vi "Roller Loop.vi"   [LabVIEW 2014]
uses:
  Common Code/Roller Indicators.ctl
  Common Code/Roller Mode Enum.ctl
  Common Code/Auto Roller Commands.ctl
  Common Code/Inner Roller States.ctl
  Sensors/Pot Data.ctl
  Untip Can States.ctl
  Roller Modes.ctl
  Really Real Manual Align.ctl
  Common Code/Change Detect Int.vi
  Robot Global Data.vi
  <vilib>/Rock Robotics/WPI/Solenoid/Deprecated/WPI_SolenoidSetBool.vi
types:
  T1 = typedef "Roller Modes.ctl" = cluster{"Auto Roller Command":T2, "Roller Mode":T3, "Override Intake Speed":dbl}
  T2 = typedef "Auto Roller Commands.ctl" = enum16{"Drag Tote", "Grab Tote", "Idle", "Eject Tote", "Untip Can", "Grab Can"}
  T3 = typedef "Roller Mode Enum.ctl" = enum16{"Manual", "Safe", "Auto"}
  T4 = typedef "Inner Roller States.ctl" = enum16{"Turn Tote Portrait", "Acquire Tote", "Absorb Tote", "Turn Tote Right", "Turn Tote Left", "Acquire Can", "Absorb Can", "Turn Can", "Hold Tote"}
  T5 = typedef "Roller Indicators.ctl" = cluster{"Rollers Closed?":bool, "Roller Mode":T3, "Auto Roller State":T2, "Tote Inside?":bool, "Intake State":T4, "Left Ping Dist":sgl, "Right Ping Dist":sgl, "Potentiometer Cluster":T6, "PING Decision":T4, "Left Arm Closed?":bool, "Portrait?":bool, "Right Arm Closed?":bool, "Left Out":sgl, "Right Out":sgl, "Left Current":sgl, "Right Current":sgl, "Tote Load Complete?":bool, "Untip Complete?":bool, "Untip State":T7, "Roller Safety Open":bool}
  T6 = typedef "Pot Data.ctl" = cluster{"Left Pot Zero":sgl, "Right Pot Zero":sgl, "Left Potentiometer":sgl, "Right Potentiometer":sgl, "Left Pot Non Zero":sgl, "Right Pot Non Zero":sgl}
  T7 = typedef "Untip Can States.ctl" = enum16{"Release Can", "Catch Can", "Idle"}
  T8 = typedef "Dashboard Control Data.ctl" = cluster{"Cam Exposure":dbl, "Go to angle":dbl, "Steer PID Gains":cluster{"proportional gain (Kc)":dbl, "integral time (Ti, min)":dbl, "derivative time (Td, min)":dbl}, "Steer PID output Range":cluster{"output high":dbl, "output low":dbl}, "Pressure m \nValue":dbl, "Pressure b \nValue":dbl, "Roller Command Cluster ":T9, "Elevator":T10, "Encoder Control":T12, "Auton Settings":cluster{"Drive Dist Window Size":dbl}, "Drivetrain Settings":T13, "Lance":T14}
  T9 = typedef "Roller Control.ctl" = cluster{"Intake Speed":dbl, "Turn In Speed":dbl, "Unload Speed":dbl, "Turn Out Speed":dbl, "Ping Align Tolerance":dbl, "Tote Range Threshold":dbl, "Right Pot 0":dbl, "Pot Threshold":dbl, "Left Pot 0":dbl, "Right Pot Scale":dbl, "Left Pot Scale":dbl, "Min Elevator Height":dbl, "Eject Time":dbl, "Eject US Threshold":dbl, "Anti-Twitch Time":u32, "Ping Caring Threshold":dbl, "Pot Diff Threshold":dbl, "Pinch Sustain":u32, "Absorb Give Up Threshold":dbl, "Untip In Threshold":dbl, "Untip Grab Range":dbl, "Ultrasonic Hold Time":u32, "Landscape Absorb Time":u32, "Pot Use Wait Time":u32, "Can Turn Stop Range":dbl, "HP Load Speed":dbl, "Stick Multiplier":dbl, "Coop Eject Speed":dbl}
  T10 = typedef "Elevator DB Control.ctl" = cluster{"PID Output Range":cluster{"output high":dbl, "output low":dbl}, "PID gains":cluster{"proportional gain (Kc)":dbl, "integral time (Ti, min)":dbl, "derivative time (Td, min)":dbl}, "Height Tolerance":sgl, " Encoder Constant":dbl, "Eject Time":sgl, "Zeroing Speed":sgl, "Presets":T11, "Ping Detect Threshold":sgl, "Trashcan Detect Threshold":sgl, "Zero Filter Time":dbl, "Stabilizer Open Time":dbl, "Zero Creep Speed":dbl, "Max Current":dbl, "Current Trip Time":dbl, "Abort Pitch":dbl, "Finger m":dbl, "Finger b":dbl, "Finger max ":dbl, "Finger Stabilizer":dbl, "Finger Store":dbl, "Finger Stop Store":dbl, "Stabilizer Close Time":dbl, "Finger min":dbl, "Unstick gain":dbl, "Full Detect Max":dbl}
  T11 = typedef "Elevator Presets.ctl" = cluster{"Pickup 2 w/ Tote":sgl, "Pickup 2 w/ Trashcan":sgl, "Pickup 3 w/ Tote":sgl, "Pickup 3 w/ Trashcan":sgl, "Bottom":sgl, "Pickup 1 w/ Tote":sgl, "Pickup Trashcan":sgl, "Pickup 1 w/ Trashcan":sgl, "Eject":sgl, "Hold Low":sgl, "Step add height":sgl, "Untip Lift":dbl, "Drop Stack":dbl, "HP Load Hold":dbl, "HP Load Drop":dbl, "HP Load Hold Can":dbl, "Store can max":dbl, "HP Drag Score":dbl, "HP Drag Finish":dbl, "Finger trashcan avoid":dbl, "Full":dbl}
  T12 = typedef "Encoder Control.ctl" = cluster{"Left Tick Constant":dbl, "Right Tick Constant":dbl, "Center Tick Constant":dbl, "Reset?":bool, "Y Dist":cluster{"PID gains":cluster{"proportional gain (Kc)":dbl, "integral time (Ti, min)":dbl, "derivative time (Td, min)":dbl}}, "X Dist":cluster{"PID gains":cluster{"proportional gain (Kc)":dbl, "integral time (Ti, min)":dbl, "derivative time (Td, min)":dbl}}, "Y Stop Thresh":dbl, "Y Stop Speed":dbl, "X Stop Thresh":dbl, "X Stop Speed":dbl}
  T13 = typedef "Drivetrain Settings.ctl" = cluster{"Gyro Tolerance":sgl, "Strafe Correct max steer":sgl, "Strafe Timer Wait":sgl, "Throttle Ramp (ms)":sgl, "Strafe Ramp (ms)":sgl, "Angular rate compensation":bool, "Throttle to Rate Scale":sgl, "Rate compensation gain":sgl, "Creep Steer":sgl, "Creep Throttle":sgl}
  T14 = typedef "Pike DB Controls.ctl" = cluster{"Down Speed":dbl, "Up Speed":dbl, "Max Down Time":dbl, "Max Up Time":dbl, "Current Limit":dbl}
  T15 = typedef "Ultrasonic Indicators.ctl" = cluster{"Left Distance":dbl, "Right Distance":dbl, "Center Distance":dbl, "Left Distance Unfilter":dbl, "Right Distance Unfilter":dbl, "Center Distance Unfilter":dbl}
  T16 = typedef "Roller Manual Bools.ctl" = cluster{"Manual Claw":bool, "Manual Align":T17, "Left Speed":dbl, "Right Speed":dbl}
  T17 = typedef "Really Real Manual Align.ctl" = enum16{"In", "Left", "Right", "Out", "Idle", "HP Load", "Speeds"}
  T18 = typedef "Elevator Status.ctl" = cluster{"Height":dbl, "Enc Value":dbl, "Limit Override":bool, "Mode":T19, "High IR":bool, "Motor Out":dbl, "Ping Detect":bool, "Auto Elevator Indicators":T20, "Master Current":dbl, "Slave Current":dbl, "High Current":bool, "Current Tripped":bool, "Top Limit":bool, "Bottom Limit":bool, "Eject Piston":bool, "Stabilizer":bool, "Finger":bool, "Finger Height":dbl, "Finger Raw":dbl, "Finger at Bottom":bool}
  T19 = typedef "Elevator Mode.ctl" = enum16{"Manual", "Safe", "Auto"}
  T20 = typedef "Auto Elevator Indicators.ctl" = cluster{"Target Out":dbl, "Storing Trashcan?":bool, "State":T21, "In Range":bool, "Store Can Command":bool, "HP Load":bool}
  T21 = typedef "Elevator State.ctl" = enum16{"Idle", "Goto Load Position", "Wait for Load", "Load Drop", "Load Lift", "Drop Stack", "Goto Eject Position", "Eject ", "Raise Trashcan", "Open Stabilizer", "Untip Drop", "Untip Wait", "Untip Lift", "Abort Load", "HP Load Wait", "HP Load Drop", "HP Load Lift", "HP Load Abort", "Close Stabilizer", "HP Load Unfinish", "HP Load Score", "HP Load Finish", "HP Goto Finish Down", "HP Goto Finish Up", "Full"}
  T22 = typedef "WPI_MotorControlDeviceRef.ctl" = cluster{"DeviceStatus":errorcluster, "Type":T23, "PWM":cluster{"Controller":T24, "PWM Channel":T25, "DeadBand":T26}, "CAN":cluster{"Device Number":u8, "Control Mode":T27, "Semaphore":T28, "Max Vout":dbl, "TalonSRX Control Mode":T29}, "Invert":bool, "TransformRef":T30, "InvTransformRef":T30}
  T23 = typedef "WPI_MotorControlType.ctl" = enum16{"PWM", "CAN", "CANTalonSRX"}
  T24 = typedef "FPGA_TypedefDigitalModule.ctl" = enum16{"Controller 1"}
  T25 = typedef "FPGA_DIOPWMChannel.ctl" = enum8{"PWM 0", "PWM 1", "PWM 2", "PWM 3", "PWM 4", "PWM 5", "PWM 6", "PWM 7", "PWM 8", "PWM 9", "PWM MXP 0", "PWM MXP 1", "PWM MXP 2", "PWM MXP 3", "PWM MXP 4", "PWM MXP 5", "PWM MXP 6", "PWM MXP 7", "PWM MXP 8", "PWM MXP 9", "Invalid"}
  T26 = typedef "WPI_PWMDeadband.ctl" = cluster{"Name":string, "maxPositivePwm":i32, "minPositivePwm":i32, "centerPwm":i32, "maxNegativePwm":i32, "minNegativePwm":i32, "angularRange":u16}
  T27 = typedef "WPI_CANJaguar_ControlMode.ctl" = enum8{"Percent VBus", "Current", "Speed", "Position", "Voltage"}
  T28 = typedef "Semaphore RefNum" = refnum<k1>
  T29 = typedef "WPI_CANTalonSRX_APIControlMode.ctl" = enum8{"Percent VBus", "Speed", "Position", "Slave", "Unchanged / Invalid"}
  T30 = typedef "WPI_PWMTransform_ConPane.ctl" = refnum<vi>
  T31 = typedef "WPI_SolenoidDevRef.ctl" = cluster{"DevStatus":errorcluster, "Pneumatics Control Module":u8, "Forward Solenoid Channel":T32, "Reverse Solenoid Channel":T32}
  T32 = typedef "WPI_SolenoidChannel.ctl" = enum8{"Solenoid 0", "Solenoid 1", "Solenoid 2", "Solenoid 3", "Solenoid 4", "Solenoid 5", "Solenoid 6", "Solenoid 7", "Invalid"}
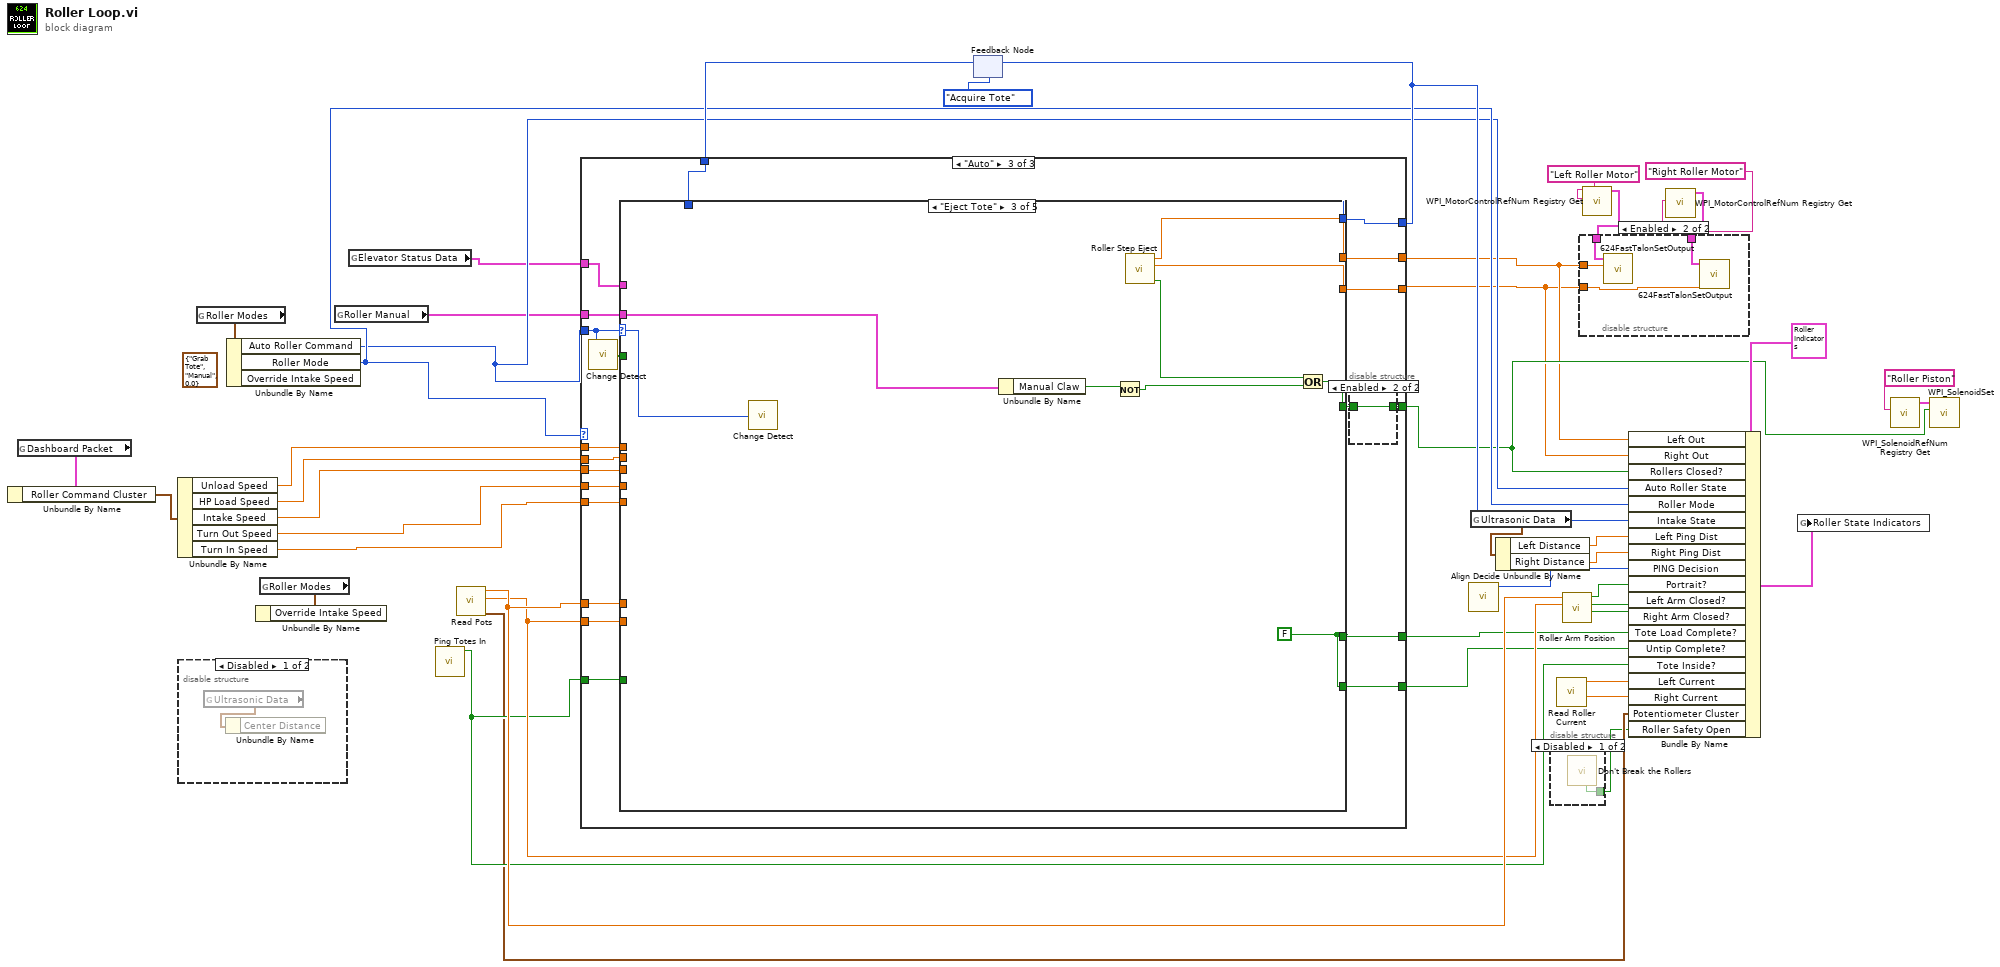
[diagram p0: block diagram]
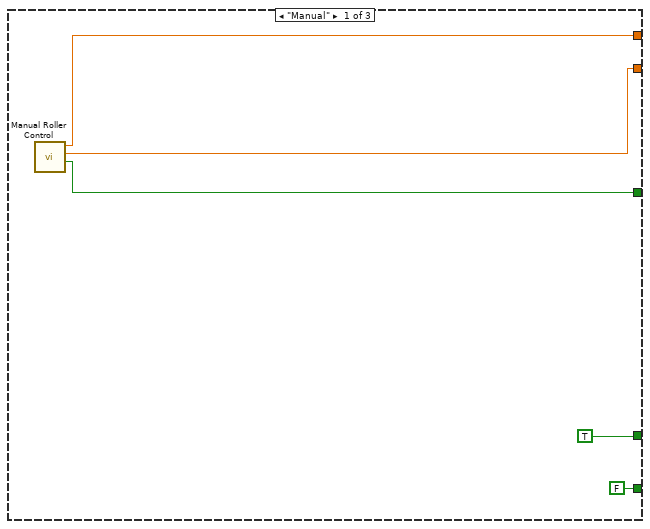
[diagram p3: hidden frame]
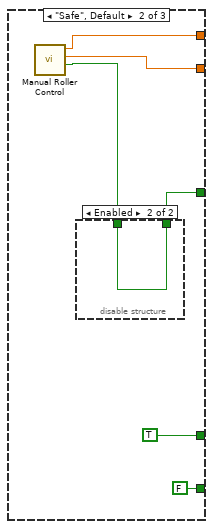
[diagram p4: hidden frame]
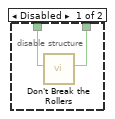
[diagram p5: hidden frame]
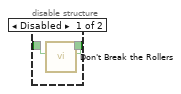
[diagram p6: hidden frame]
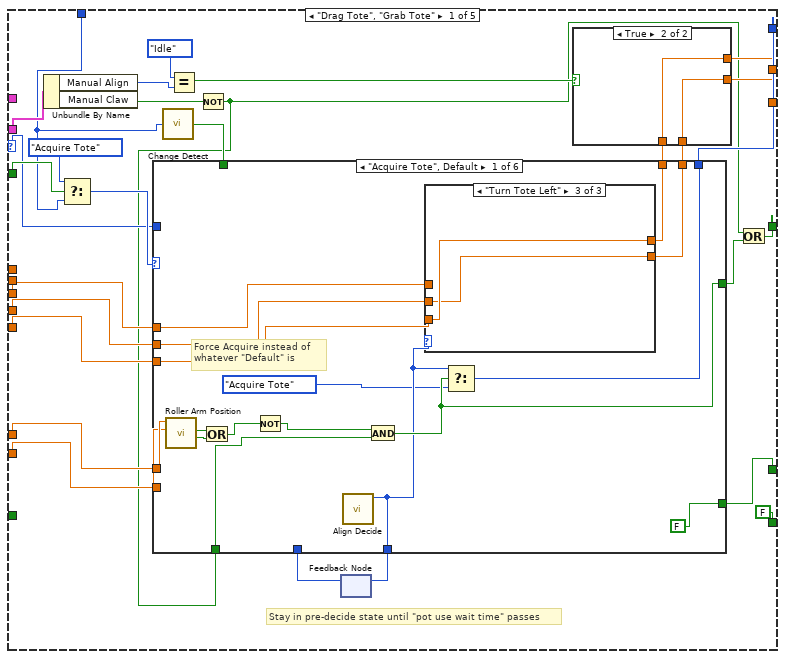
[diagram p7: hidden frame]
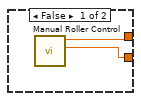
[diagram p8: hidden frame]
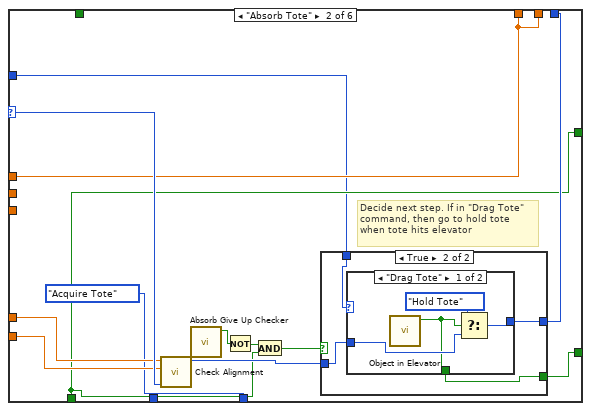
[diagram p11: hidden frame]
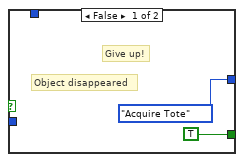
[diagram p12: hidden frame]
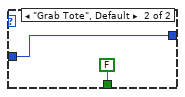
[diagram p13: hidden frame]
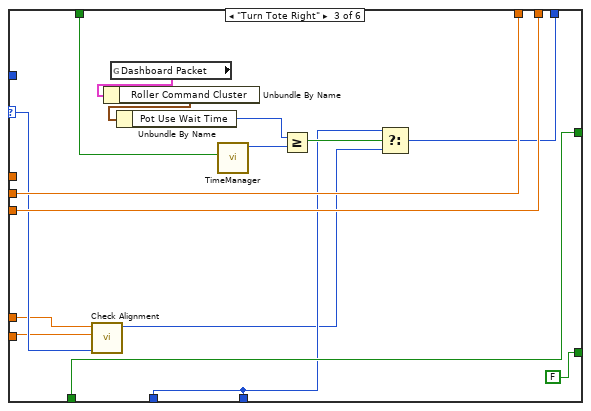
[diagram p14: hidden frame]
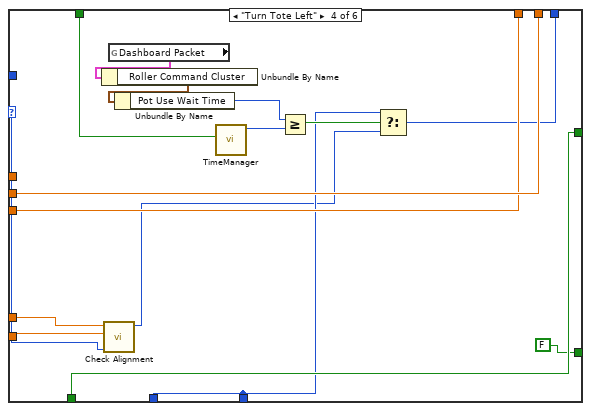
[diagram p15: hidden frame]
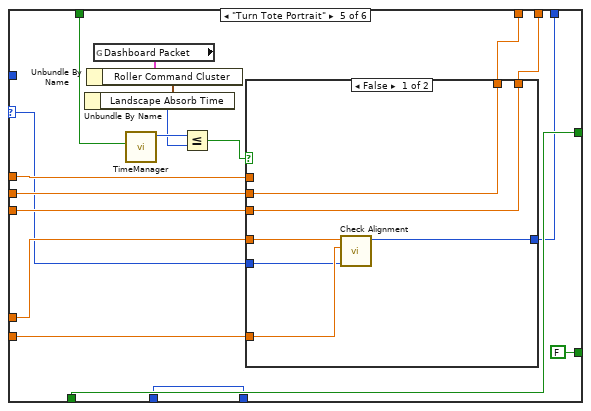
[diagram p16: hidden frame]
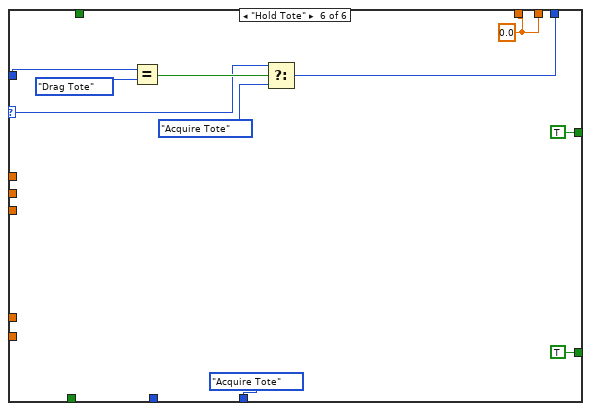
[diagram p18: hidden frame]
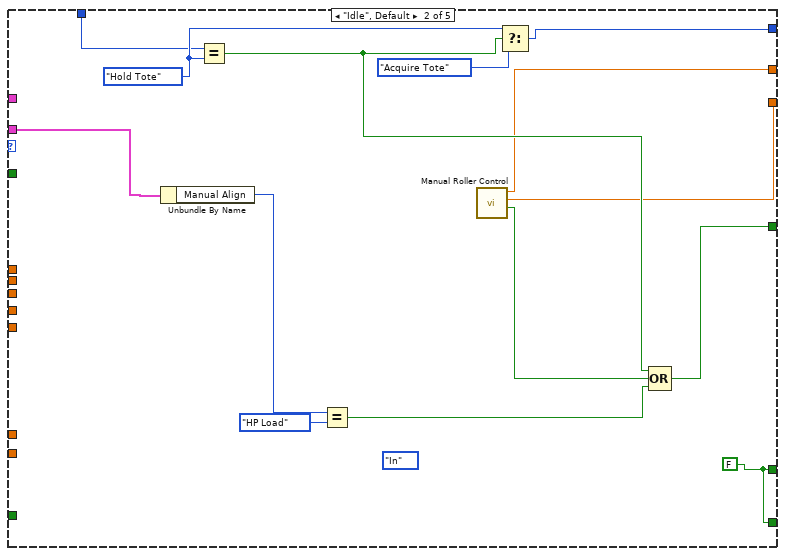
[diagram p19: hidden frame]
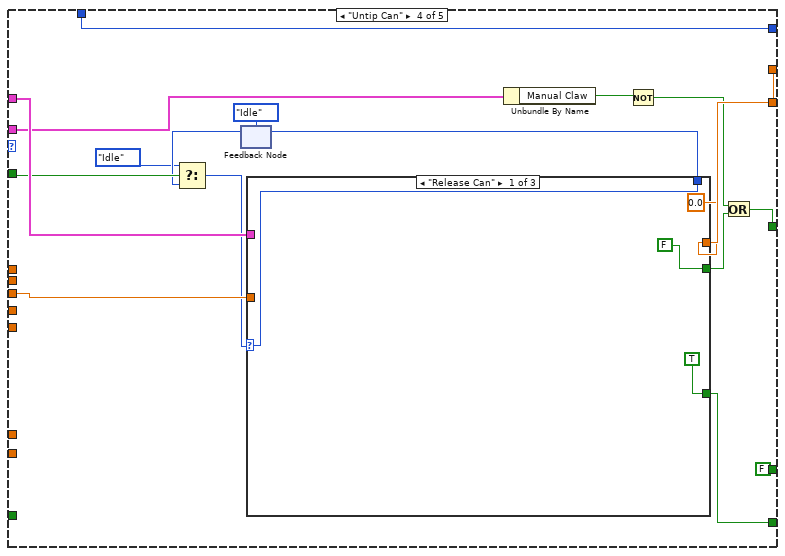
[diagram p20: hidden frame]
diagram:
  (unwired) T1 {"Auto Roller Command"=enum."Grab Tote", "Roller Mode"=enum."Manual", "Override Intake Speed"=0.0} ("input cluster")
  n1 = global read "Robot Global Data.vi" "Dashboard Packet"() -> (w24:T8)
  n2 = Unbundle By Name(w24) -> ("Roller Command Cluster"=w25:T9)
  n3 = Unbundle By Name(w25) -> ("Unload Speed"=w12:dbl, "HP Load Speed"=w4:dbl, "Intake Speed"=w11:dbl, "Turn Out Speed"=w2:dbl, "Turn In Speed"=w1:dbl)
  n4 = disable-structure shown="Disabled" {
    frame Disabled {
      n5 = global read "Robot Global Data.vi" "Ultrasonic Data"() -> (w44:T15)
      n6 = Unbundle By Name(w44) -> ()  [unwired: 1 out]
    }
    frame Enabled {
    }
  }
  n7 = global read "Robot Global Data.vi" "Roller Modes"() -> (w38:T1)
  n8 = Unbundle By Name(w38) -> ("Auto Roller Command"=w35:T2, "Roller Mode"=w36:T3)  [unwired: 1 out]
  n9 = global read "Robot Global Data.vi" "Roller Modes"() -> (w3:T1)
  n10 = Unbundle By Name(w3) -> ()  [unwired: 1 out]
  n11 = global read "Robot Global Data.vi" "Roller Manual"() -> (w20:T16)
  n12 = global read "Robot Global Data.vi" "Elevator Status Data"() -> (w21:T18)
  n13 = call "Ping Totes In.vi"() -> ("In?"=w10:bool)  [unwired: 11 in]
  n14 = call "Read Pots.vi"() -> ("Pot Write Cluster"=w7:T6, "Right Pot"=w28:dbl, "Left Pot"=w29:dbl)  [unwired: 7 in, 2 out]
  n15 = feedback #1(Inner_Roller_States."Acquire Tote" ("Enum")) -> (w42:T4)
  n16 = case shown="\"Auto\"" w36 {
    tunnel: w20 -> [_ _ w69]
    tunnel: w11 -> [_ _ w77]
    tunnel: w2 -> [_ _ w75]
    tunnel: w1 -> [_ _ w76]
    tunnel: w35 -> [_ _ w60]
    tunnel: [_ _ w73] -> w37
    tunnel: w42 -> [_ _ w78]
    tunnel: [w45 w55 w66] -> w33
    tunnel: w10 -> [_ _ w74]
    tunnel: [w47 w52 w72] -> w27
    tunnel: [w46 w51 w71] -> w26
    tunnel: w12 -> [_ _ w70]
    tunnel: w29 -> [_ _ w68]
    tunnel: w28 -> [_ _ w67]
    tunnel: [TRUE TRUE w64] -> w23
    tunnel: w21 -> [_ _ w63]
    tunnel: [FALSE FALSE w61] -> w22
    tunnel: w4 -> [_ _ w59]
    frame "Manual" {
      n17 = call "Manual Roller Control.vi"() -> ("Boolean"=w45:bool, "Right Speed Out"=w46:dbl, "Left Speed Out"=w47:dbl)  [unwired: 9 in]
    }
    frame "Safe", Default {
      n18 = call "Manual Roller Control.vi"() -> ("Boolean"=w50:bool, "Right Speed Out"=w51:dbl, "Left Speed Out"=w52:dbl)  [unwired: 9 in]
      n19 = disable-structure shown="Enabled" {
        disable-tunnel: [w57 w58] -> w55
        disable-tunnel: w50 -> [w56 w58]
        frame Disabled {
          n20 = call "Don't Break the Rollers.vi"("Rollers close in"=w56) -> ("Roller close out"=w57:bool)  [unwired: 9 in, 1 out]
        }
        frame Enabled {
        }
      }
    }
    frame "Auto" {
      n21 = call-poly "Change Detect.vi"("In"=w60) -> ("Changed?"=w62:bool)
      n22 = case shown="\"Eject Tote\"" w60 {
        selector: w60 -> [w85 _ w250 _ _]
        tunnel: w78 -> [w88 w237 w252 w267 w320]
        tunnel: [w84 w238 w247 w257 w302] -> w65
        tunnel: w77 -> [w109 _ _ w265 w316]
        tunnel: w76 -> [w108 _ _ _ w314]
        tunnel: w75 -> [w107 _ _ _ w315]
        tunnel: w74 -> [_ _ _ _ _]
        tunnel: [w97 w236 w252 w267 w311] -> w73
        tunnel: [w96 w231 w249 w260 w312] -> w72
        tunnel: [w93 w230 w248 w260 w313] -> w71
        tunnel: w70 -> [_ _ _ _ _]
        tunnel: w69 -> [w103 w242 w244 w254 w322]
        tunnel: w68 -> [w106 _ _ _ _]
        tunnel: w67 -> [w105 _ _ _ _]
        tunnel: [w104 w241 w251 FALSE FALSE] -> w64
        tunnel: w63 -> [_ _ _ w268 _]
        tunnel: w62 -> [w89 _ _ w264 w321]
        tunnel: [FALSE w241 w251 w259 FALSE] -> w61
        tunnel: w59 -> [_ _ _ _ _]
        frame "Drag Tote", "Grab Tote" {
          # "Stay in pre-decide state until \"pot use wait time\" passes"
          n23 = Unbundle By Name(w103) -> ("Manual Align"=w100:T17, "Manual Claw"=w102:bool)
          n24 = Select(t=Inner_Roller_States."Acquire Tote", s=w89, f=w88) -> (s? t:f=w86:T4)
          n25 = call-poly "Change Detect.vi"("In"=w88) -> ("Changed?"=w92:bool)
          n26 = Equal?(x=Really_Real_Manual_Align."Idle" ("y"), y=w100) -> (x = y?=w98:bool)
          n27 = Not(x=w102) -> (.not. x?=w82:bool)
          n28 = feedback #2() -> (w90:T4)  [unwired: 1 in]
          n29 = case shown="\"Acquire Tote\", Default" w86 {
            selector: w86 -> [_ w146 w174 w192 w198 w221]
            tunnel: w82 -> [w120 w140 w171 w187 w204 _]
            tunnel: [w119 w140 w171 w187 w204 TRUE] -> w83
            tunnel: [w130 w148 w161 w179 w197 w219] -> w97
            tunnel: w109 -> [w129 w143 _ _ w207 _]
            tunnel: w108 -> [w128 _ w176 w188 w201 _]
            tunnel: w107 -> [w127 _ w175 w189 w202 _]
            tunnel: [w126 w143 w175 w188 w206 w228] -> w95
            tunnel: [w125 w143 w176 w189 w205 w228] -> w94
            tunnel: w106 -> [w124 w145 w173 w191 w199 _]
            tunnel: w105 -> [w123 w144 w172 w190 w200 _]
            tunnel: [FALSE w142 FALSE FALSE FALSE TRUE ("Boolean")] -> w104
            tunnel: w92 -> [_ _ w167 w182 w210 _]
            tunnel: [w115 Inner_Roller_States."Acquire Tote" ("Next Step") w163 w181 w193 Inner_Roller_States."Acquire Tote" ("Next Step")] -> w91
            tunnel: w90 -> [_ _ w163 w181 w193 _]
            tunnel: w85 -> [_ w136 _ _ _ w224]
            frame "Acquire Tote", Default {
              # "Force Acquire instead of \nwhatever \"Default\" is"
              n30 = call "Roller Arm Position.vi"("Right Pot"=w123, "Left Pot"=w124) -> ("Right Closed?"=w122:bool, "Left Closed?"=w121:bool)  [unwired: 6 in, 2 out]
              n31 = Or(x=w121, y=w122) -> (x .or. y?=w118:bool)
              n32 = Not(x=w118) -> (.not. x?=w117:bool)
              n33 = call "Align Decide.vi"() -> ("Next Step"=w115:T4)  [unwired: 11 in]
              n34 = And(x=w117, y=w120) -> (x .and. y?=w119:bool)
              n35 = case shown="\"Turn Tote Left\"" w115 {
                tunnel: w129 -> [w131 _ _]
                tunnel: w128 -> [_ w133 w135]
                tunnel: w127 -> [_ w132 w134]
                tunnel: [w131 w132 w135] -> w126
                tunnel: [w131 w133 w134] -> w125
                frame "Absorb Tote", Default {
                }
                frame "Turn Tote Right" {
                }
                frame "Turn Tote Left" {
                }
              }
              n36 = Select(t=w115, s=w119, f=Inner_Roller_States."Acquire Tote") -> (s? t:f=w130:T4)
            }
            frame "Absorb Tote" {
              # "Decide next step. If in \"Drag Tote\"\ncommand, then go to hold tote\nwhen tote hits elevator"
              n37 = call "Check Alignment.vi"("Current State"=w146, "Right Pot"=w144, "Left Pot"=w145) -> ("State Output"=w147:T4)  [unwired: 8 in]
              n38 = call "Absorb Give Up Checker.vi"() -> ("Give Up?"=w141:bool)  [unwired: 11 in]
              n39 = Not(x=w141) -> (.not. x?=w139:bool)
              n40 = And(x=w139, y=w140) -> (x .and. y?=w138:bool)
              n41 = case shown="True" w138 {
                tunnel: [Inner_Roller_States."Acquire Tote" ("State Output") w152] -> w148
                tunnel: w147 -> [_ w153]
                tunnel: [TRUE w151] -> w142
                tunnel: w136 -> [_ w154]
                frame False {
                  # "Object disappeared"
                  # "Give up!"
                }
                frame True {
                  n42 = case shown="\"Drag Tote\"" w154 {
                    tunnel: w153 -> [w158 w160]
                    tunnel: [w157 w160] -> w152
                    tunnel: [w155 FALSE ("Boolean")] -> w151
                    frame "Drag Tote" {
                      n43 = call "Object in Elevator.vi"() -> ("Ping Detect"=w155:bool)  [unwired: 11 in]
                      n44 = Select(t=Inner_Roller_States."Hold Tote", s=w155, f=w158) -> (s? t:f=w157:T4)
                    }
                    frame "Grab Tote", Default {
                    }
                  }
                }
              }
            }
            frame "Turn Tote Right" {
              n45 = call "Check Alignment.vi"("Current State"=w174, "Right Pot"=w172, "Left Pot"=w173) -> ("State Output"=w162:T4)  [unwired: 8 in]
              n46 = global read "Robot Global Data.vi" "Dashboard Packet"() -> (w169:T8)
              n47 = Unbundle By Name(w169) -> ("Roller Command Cluster"=w168:T9)
              n48 = Unbundle By Name(w168) -> ("Pot Use Wait Time"=w165:u32)
              n49 = call "TimeManager.vi"("Reset?"=w167) -> ("Time Since Reset"=w166:u32)  [unwired: 9 in, 1 out]
              n50 = Greater Or Equal?(x=w165, y=w166) -> (x >= y?=w164:bool)
              n51 = Select(t=w163, s=w164, f=w162) -> (s? t:f=w161:T4)
            }
            frame "Turn Tote Left" {
              n52 = call "Check Alignment.vi"("Current State"=w192, "Right Pot"=w190, "Left Pot"=w191) -> ("State Output"=w180:T4)  [unwired: 8 in]
              n53 = global read "Robot Global Data.vi" "Dashboard Packet"() -> (w177:T8)
              n54 = Unbundle By Name(w177) -> ("Roller Command Cluster"=w178:T9)
              n55 = Unbundle By Name(w178) -> ("Pot Use Wait Time"=w184:u32)
              n56 = call "TimeManager.vi"("Reset?"=w182) -> ("Time Since Reset"=w183:u32)  [unwired: 9 in, 1 out]
              n57 = Greater Or Equal?(x=w184, y=w183) -> (x >= y?=w185:bool)
              n58 = Select(t=w181, s=w185, f=w180) -> (s? t:f=w179:T4)
            }
            frame "Turn Tote Portrait" {
              n59 = global read "Robot Global Data.vi" "Dashboard Packet"() -> (w196:T8)
              n60 = Unbundle By Name(w196) -> ("Roller Command Cluster"=w195:T9)
              n61 = Unbundle By Name(w195) -> ("Landscape Absorb Time"=w194:u32)
              n62 = call "TimeManager.vi"("Reset?"=w210) -> ("Time Since Reset"=w209:u32)  [unwired: 9 in, 1 out]
              n63 = Less Or Equal?(x=w209, y=w194) -> (x <= y?=w208:bool)
              n64 = case shown="False" w208 {
                tunnel: [w216 w218] -> w206
                tunnel: w207 -> [_ w218]
                tunnel: [w215 w218] -> w205
                tunnel: w202 -> [w216 _]
                tunnel: w201 -> [w215 _]
                tunnel: w200 -> [w214 _]
                tunnel: w199 -> [w213 _]
                tunnel: w198 -> [w212 w217]
                tunnel: [w211 w217] -> w197
                frame False {
                  n65 = call "Check Alignment.vi"("Current State"=w212, "Right Pot"=w214, "Left Pot"=w213) -> ("State Output"=w211:T4)  [unwired: 8 in]
                }
                frame True {
                }
              }
            }
            frame "Hold Tote" {
              w228 = 0.0
              n66 = Equal?(x=w224, y=Auto_Roller_Commands."Drag Tote") -> (x = y?=w222:bool)
              n67 = Select(t=w221, s=w222, f=Inner_Roller_States."Acquire Tote") -> (s? t:f=w219:T4)
            }
          }
          n68 = feedback-in #2(w91) -> ()
          n69 = case shown="True" w98 {
            tunnel: [w111 w113] -> w96
            tunnel: w95 -> [_ w113]
            tunnel: [w110 w112] -> w93
            tunnel: w94 -> [_ w112]
            frame False {
              n70 = call "Manual Roller Control.vi"() -> ("Right Speed Out"=w110:dbl, "Left Speed Out"=w111:dbl)  [unwired: 9 in, 1 out]
            }
            frame True {
            }
          }
          n71 = Or(x=w82, y=w83) -> (x .or. y?=w84:bool)
        }
        frame "Idle", Default {
          (unwired) Really_Real_Manual_Align."In" ("Manual Align")
          w240 = Inner_Roller_States."Hold Tote" ("y")
          w241 = FALSE
          n72 = Unbundle By Name(w242) -> ("Manual Align"=w234:T17)
          n73 = Equal?(x=w237, y=w240) -> (x = y?=w239:bool)
          n74 = Equal?(x=w234, y=Really_Real_Manual_Align."HP Load") -> (x = y?=w232:bool)
          n75 = call "Manual Roller Control.vi"() -> ("Boolean"=w229:bool, "Right Speed Out"=w230:dbl, "Left Speed Out"=w231:dbl)  [unwired: 9 in]
          n76 = Select(t=w240, s=w239, f=Inner_Roller_States."Acquire Tote") -> (s? t:f=w236:T4)
          n77 = Compound Arithmetic op=OR(w239, w229, w232) -> (w238:bool)
        }
        frame "Eject Tote" {
          w251 = FALSE
          n78 = call-poly "Change Detect.vi"("In"=w250) -> ()  [unwired: 1 out]
          n79 = Unbundle By Name(w244) -> ("Manual Claw"=w245:bool)
          n80 = Not(x=w245) -> (.not. x?=w246:bool)
          n81 = call "Roller Step Eject.vi"() -> ("Close Rollers?"=w243:bool, "Right Out"=w248:dbl, "Left Out"=w249:dbl)  [unwired: 9 in]
          n82 = Or(x=w243, y=w246) -> (x .or. y?=w247:bool)
        }
        frame "Untip Can" {
          n83 = feedback #3(Untip_Can_States."Idle") -> (w263:T7)
          n84 = Select(t=Untip_Can_States."Idle", s=w264, f=w263) -> (s? t:f=w262:T7)
          n85 = case shown="\"Release Can\"" w262 {
            selector: w262 -> [w270 w281 w295]
            tunnel: w268 -> [_ _ w291]
            tunnel: w265 -> [_ w284 w298]
            tunnel: [0.0 ("Intake Speed") w284 w298] -> w260
            tunnel: [FALSE TRUE FALSE] -> w253
            tunnel: [TRUE FALSE FALSE] -> w259
            tunnel: [w270 w280 w294] -> w258
            frame "Release Can" {
            }
            frame "Catch Can" {
              n86 = global read "Robot Global Data.vi" "Dashboard Packet"() -> (w277:T8)
              n87 = global read "Robot Global Data.vi" "Ultrasonic Data"() -> (w275:T15)
              n88 = Unbundle By Name(w275) -> ("Center Distance"=w276:dbl)
              n89 = Unbundle By Name(w277) -> ("Roller Command Cluster.Untip In Threshold"=w278:dbl)
              n90 = Less Or Equal?(x=w276, y=w278) -> (x <= y?=w279:bool)
              n91 = Select(t=Untip_Can_States."Release Can", s=w279, f=w281) -> (s? t:f=w280:T7)
            }
            frame "Idle", Default {
              n92 = global read "Robot Global Data.vi" "Dashboard Packet"() -> (w286:T8)
              n93 = global read "Robot Global Data.vi" "Ultrasonic Data"() -> (w288:T15)
              n94 = Unbundle By Name(w286) -> ("Roller Command Cluster.Untip Grab Range"=w287:dbl)
              n95 = Unbundle By Name(w288) -> ("Center Distance"=w289:dbl)
              n96 = Unbundle By Name(w291) -> ("Auto Elevator Indicators.In Range"=w292:bool)
              n97 = Less Or Equal?(x=w289, y=w287) -> (x <= y?=w290:bool)
              n98 = And(x=w292, y=w290) -> (x .and. y?=w293:bool)
              n99 = Select(t=Untip_Can_States."Catch Can", s=w293, f=w295) -> (s? t:f=w294:T7)
            }
          }
          n100 = feedback-in #3(w258) -> ()
          n101 = Unbundle By Name(w254) -> ("Manual Claw"=w255:bool)
          n102 = Not(x=w255) -> (.not. x?=w256:bool)
          n103 = Or(x=w256, y=w253) -> (x .or. y?=w257:bool)
        }
        frame "Grab Can" {
          n104 = Unbundle By Name(w322) -> ("Manual Align"=w317:T17, "Manual Claw"=w299:bool)
          n105 = global read "Robot Global Data.vi" "Dashboard Packet"() -> (w306:T8)
          n106 = global read "Robot Global Data.vi" "Ultrasonic Data"() -> (w307:T15)
          n107 = Unbundle By Name(w307) -> ("Center Distance"=w305:dbl)
          n108 = Unbundle By Name(w306) -> ("Roller Command Cluster.Can Turn Stop Range"=w304:dbl)
          n109 = Not(x=w299) -> (.not. x?=w300:bool)
          n110 = Select(t=Inner_Roller_States."Acquire Can", s=w321, f=w320) -> (s? t:f=w318:T4)
          n111 = Less Or Equal?(x=w305, y=w304) -> (x <= y?=w303:bool)
          n112 = Or(x=w300, y=w303) -> (x .or. y?=w310:bool)
          n113 = case shown="\"Absorb Can\"" w318 {
            selector: w318 -> [w325 w331 w340]
            tunnel: w317 -> [_ _ w341]
            tunnel: [w327 w332 w336] -> w312
            tunnel: w316 -> [w327 w332 w334]
            tunnel: w315 -> [_ _ w337]
            tunnel: w314 -> [_ _ w335]
            tunnel: [w327 w332 w338] -> w313
            tunnel: [w324 w329 w339] -> w311
            tunnel: w310 -> [w326 w328 _]
            tunnel: [w326 w328 TRUE] -> w301
            frame "Absorb Can" {
              n114 = Select(t=w325, s=w326, f=Inner_Roller_States."Acquire Can") -> (s? t:f=w324:T4)
            }
            frame "Acquire Can", Default {
              n115 = Select(t=Inner_Roller_States."Turn Can", s=w328, f=w331) -> (s? t:f=w329:T4)
            }
            frame "Turn Can" {
              n116 = case shown="Default" w341 {
                tunnel: w340 -> [_ w346 w349 w350]
                tunnel: [Inner_Roller_States."Absorb Can" ("t") w346 w349 w350] -> w339
                tunnel: [w342 w345 w347 w351] -> w338
                tunnel: w337 -> [_ w345 w348 _]
                tunnel: [w342 w344 w348 w351] -> w336
                tunnel: w335 -> [_ w344 w347 _]
                tunnel: w334 -> [w342 _ _ _]
                frame "In" {
                }
                frame "Left" {
                }
                frame "Right" {
                }
                frame Default {
                  w351 = 0.0
                }
              }
            }
          }
          n117 = Or(x=w301, y=w300) -> (x .or. y?=w302:bool)
        }
      }
      n118 = disable-structure shown="Enabled" {
        disable-tunnel: [w80 w81] -> w66
        disable-tunnel: w65 -> [w79 w81]
        frame Disabled {
          n119 = call "Don't Break the Rollers.vi"("Rollers close in"=w79) -> ("Roller close out"=w80:bool)  [unwired: 9 in, 1 out]
        }
        frame Enabled {
        }
      }
    }
  }
  n120 = feedback-in #1(w37) -> ()
  n121 = call "Align Decide.vi"() -> ("Next Step"=w34:T4)  [unwired: 11 in]
  n122 = global read "Robot Global Data.vi" "Ultrasonic Data"() -> (w13:T15)
  n123 = Unbundle By Name(w13) -> ("Left Distance"=w15:dbl, "Right Distance"=w14:dbl)
  n124 = disable-structure shown="Disabled" {
    disable-tunnel: [w352 _] -> w5
    frame Disabled {
      n125 = call "Don't Break the Rollers.vi"() -> ("Keeep rollers open?"=w352:bool)  [unwired: 10 in, 1 out]
    }
    frame Enabled {
    }
  }
  n126 = call "Read Roller Current.vi"() -> ("R Current"=w8:dbl, "L Current"=w9:dbl)  [unwired: 10 in]
  n127 = call "Roller Arm Position.vi"("Right Pot"=w28, "Left Pot"=w29) -> ("Right Closed?"=w30:bool, "Left Closed?"=w31:bool, "Portrait?"=w32:bool)  [unwired: 6 in, 1 out]
  n128 = call <vilib>:"WPI_MotorControlRefNum Registry Get.vi"("refnum name"="Left Roller Motor") -> ("MotorControlDevRef"=w19:T22)  [unwired: 9 in, 1 out]
  n129 = Bundle By Name(cluster=T5 {"Rollers Closed?"=FALSE, "Roller Mode"=enum."Manual", "Auto Roller State"=enum."Grab Tote", "Tote Inside?"=FALSE, "Intake State"=enum."Acquire Tote", "Left Ping Dist"=0.0, "Right Ping Dist"=0.0, "Potentiometer Cluster"={"Left Pot Zero"=0.0, "Right Pot Zero"=0.0, "Left Potentiometer"=0.0, "Right Potentiometer"=0.0, "Left Pot Non Zero"=0.0, "Right Pot Non Zero"=0.0}, "PING Decision"=enum."Acquire Tote", "Left Arm Closed?"=FALSE, "Portrait?"=FALSE, "Right Arm Closed?"=FALSE, "Left Out"=0.0, "Right Out"=0.0, "Left Current"=0.0, "Right Current"=0.0, "Tote Load Complete?"=FALSE, "Untip Complete?"=FALSE, "Untip State"=enum."Idle", "Roller Safety Open"=FALSE} ("Roller State Indicators"), "Left Out"=w27, "Right Out"=w26, "Rollers Closed?"=w33, "Auto Roller State"=w35, "Roller Mode"=w36, "Intake State"=w37, "Left Ping Dist"=w15, "Right Ping Dist"=w14, "PING Decision"=w34, "Portrait?"=w32, "Left Arm Closed?"=w31, "Right Arm Closed?"=w30, "Tote Load Complete?"=w23, "Untip Complete?"=w22, "Tote Inside?"=w10, "Left Current"=w9, "Right Current"=w8, "Potentiometer Cluster"=w7, "Roller Safety Open"=w5) -> (w41:T5)
  n130 = call <vilib>:"WPI_MotorControlRefNum Registry Get.vi"("refnum name"="Right Roller Motor") -> ("MotorControlDevRef"=w17:T22)  [unwired: 9 in, 1 out]
  n131 = disable-structure shown="Enabled" {
    disable-tunnel: w19 -> [w355 w357]
    disable-tunnel: w27 -> [w356 w360]
    disable-tunnel: w17 -> [w353 w358]
    disable-tunnel: w26 -> [w354 w359]
    frame Disabled {
      n132 = call <vilib>:"WPI_MotorControlSetOutput.vi"("Output"=w356, "MotorControlDevRef"=w355) -> ()  [unwired: 7 in, 3 out]
      n133 = call <vilib>:"WPI_MotorControlSetOutput.vi"("Output"=w354, "MotorControlDevRef"=w353) -> ()  [unwired: 7 in, 3 out]
    }
    frame Enabled {
      n134 = call "624FastTalonSetOutput.vi"("Output"=w360, "MotorControlDevRef"=w357) -> ()  [unwired: 8 in, 2 out]
      n135 = call "624FastTalonSetOutput.vi"("Output"=w359, "MotorControlDevRef"=w358) -> ()  [unwired: 8 in, 2 out]
    }
  }
  n136 = global write "Robot Global Data.vi" "Roller State Indicators"(w41) -> ()
  n137 = call <vilib>:"WPI_SolenoidRefNum Registry Get.vi"("refnum name"="Roller Piston") -> ("SolenoidDevRef"=w39:T31)  [unwired: 9 in, 1 out]
  n138 = call-poly <vilib>:"WPI_SolenoidSet.vi"("Value"=w33, "SolenoidDevRef"=w39) -> ()  [unwired: 8 in, 2 out]
